vi "Simulate Statechart.vi"(4 "C DLL path":path=path "D:/Users/jjensen/workspace/Simulated iRobot Navigation/Release/libSimulated iRobot Navigation.dll", 6 "Execution Mode":T12, 8 "stop":bool, 11 "Statechart Inputs In":T2={"net distance (mm)"=0, "net angle (deg)"=0, "Max Wheel Speed (mm/s)"=0, "accelerometer"={"x axis (g)"=0.0, "y axis (g)"=0.0, "z axis (g)"=0.0}, "iRobot Sensors"={"Bumps + Wheel Drops"={"Wheeldrop Caster"=FALSE, "Wheeldrop Left"=FALSE, "Wheeldrop Right"=FALSE, "Bump Left"=FALSE, "Bump Right"=FALSE}, "Wall"=FALSE, "Cliff Left"=FALSE, "Cliff Front Left"=FALSE, "Cliff Front Right"=FALSE, "Cliff Right"=FALSE, "Virtual Wall"=FALSE, "Low-Side Driver + Wheel Overcurrent"={"Low-Side Driver 0"=FALSE, "Low-Side Driver 1"=FALSE, "Low-Side Driver 2"=FALSE, "Left Wheel"=FALSE, "Right Wheel"=FALSE}, "Infrared"=255, "Buttons"={"Advance"=FALSE, "Play"=FALSE}, "Distance (mm)"=0, "Angle (deg)"=0, "Charging State"=enum."Not Charging", "Voltage (mV)"=0, "Current (mA)"=0, "Battery Temperature (deg C)"=0, "Battery Charge (mAh)"=0, "Battery Capacity (mAh)"=0, "Wall Signal (0-4095)"=0, "Cliff Left Signal (0-4095)"=0, "Cliff Front Left Signal (0-4095)"=0, "Cliff Front Right Signal (0-4095)"=0, "Cliff Right Signal (0-4095)"=0, "Cargo Bay Digital Inputs"={"Digital Input 0"=FALSE, "Digital Input 1"=FALSE, "Digital Input 2"=FALSE, "Digital Input 3"=FALSE, "Device Detect"=FALSE}, "Cargo Bay Analog Signal (0-1023)"=0, "Charging Sources Available"={"Internal Charger"=FALSE, "Home Base"=FALSE}, "OI Mode"=enum."Off", "Song Number"=0, "Song Playing"=FALSE, "Number of Stream Packets"=0, "Requested Velocity (mm/s)"=0, "Requested Radius (mm)"=0, "Requested Right Wheel Velocity (mm/s)"=0, "Requested Left Wheel Velocity (mm/s)"=0}, "Is Simulator?"=FALSE} {"iRobot Sensors"."Infrared" format="%02x"; "accelerometer"."z axis (g)" format="%.3f"; "accelerometer"."y axis (g)" format="%.3f"; "accelerometer"."x axis (g)" format="%.3f"; "Max Wheel Speed (mm/s)" scale=0.0..500.0}) -> (0 "Left Wheel Speed (mm/s)":i16, 1 "Right Wheel Speed (mm/s)":i16, 2 "Diagram Display":picture, 3 "Statechart Inputs Out":T2={"net distance (mm)"=0, "net angle (deg)"=0, "Max Wheel Speed (mm/s)"=0, "accelerometer"={"x axis (g)"=0.0, "y axis (g)"=0.0, "z axis (g)"=0.0}, "iRobot Sensors"={"Bumps + Wheel Drops"={"Wheeldrop Caster"=FALSE, "Wheeldrop Left"=FALSE, "Wheeldrop Right"=FALSE, "Bump Left"=FALSE, "Bump Right"=FALSE}, "Wall"=FALSE, "Cliff Left"=FALSE, "Cliff Front Left"=FALSE, "Cliff Front Right"=FALSE, "Cliff Right"=FALSE, "Virtual Wall"=FALSE, "Low-Side Driver + Wheel Overcurrent"={"Low-Side Driver 0"=FALSE, "Low-Side Driver 1"=FALSE, "Low-Side Driver 2"=FALSE, "Left Wheel"=FALSE, "Right Wheel"=FALSE}, "Infrared"=255, "Buttons"={"Advance"=FALSE, "Play"=FALSE}, "Distance (mm)"=0, "Angle (deg)"=0, "Charging State"=enum."Not Charging", "Voltage (mV)"=0, "Current (mA)"=0, "Battery Temperature (deg C)"=0, "Battery Charge (mAh)"=0, "Battery Capacity (mAh)"=0, "Wall Signal (0-4095)"=0, "Cliff Left Signal (0-4095)"=0, "Cliff Front Left Signal (0-4095)"=0, "Cliff Front Right Signal (0-4095)"=0, "Cliff Right Signal (0-4095)"=0, "Cargo Bay Digital Inputs"={"Digital Input 0"=FALSE, "Digital Input 1"=FALSE, "Digital Input 2"=FALSE, "Digital Input 3"=FALSE, "Device Detect"=FALSE}, "Cargo Bay Analog Signal (0-1023)"=0, "Charging Sources Available"={"Internal Charger"=FALSE, "Home Base"=FALSE}, "OI Mode"=enum."Off", "Song Number"=0, "Song Playing"=FALSE, "Number of Stream Packets"=0, "Requested Velocity (mm/s)"=0, "Requested Radius (mm)"=0, "Requested Right Wheel Velocity (mm/s)"=0, "Requested Left Wheel Velocity (mm/s)"=0}, "Is Simulator?"=FALSE} {"iRobot Sensors"."Infrared" format="%02x"; "accelerometer"."z axis (g)" format="%.3f"; "accelerometer"."y axis (g)" format="%.3f"; "accelerometer"."x axis (g)" format="%.3f"; "Max Wheel Speed (mm/s)" scale=0.0..500.0}, 5 "Active States":string[](array[string]))   [LabVIEW 2013]
uses:
  Simulate Execution Mode.ctl
  iRobot Navigation State Machine.lvsc/Inputs.ctl
  Accelerometer.ctl
  iRobot/Sensor/Sensor Group 6.ctl
  iRobot/Sensor/Bumps + Wheel Drops.ctl
  iRobot/Sensor/Low-Side Driver + Wheel Overcurrent.ctl
  iRobot/Sensor/Buttons.ctl
  iRobot/Sensor/Charging State.ctl
  iRobot/Sensor/Cargo Bay Digital Inputs.ctl
  iRobot/Sensor/Charging Sources Available.ctl
  iRobot/Sensor/OI Mode.ctl
  iRobot Navigation State Machine.lvsc/StatechartState.ctl
  iRobot Navigation State Machine.lvsc/State.ctl
  iRobot Navigation State Machine.lvsc/CompanionDiagram.vi/64/SC Main.vi
  iRobot Navigation State Machine.lvsc/CompanionDiagram.vi/64/Upd State.vi
  iRobot Navigation State Machine.lvsc/CompanionDiagram.vi/64/Trans Graph0.vi
  iRobot Navigation State Machine.lvsc/CompanionDiagram.vi/64/EnterGraphCore.vi
  iRobot Navigation State Machine.lvsc/CompanionDiagram.vi/64/Trans Graph1.vi
  iRobot Navigation State Machine.lvsc/CompanionDiagram.vi/64/Trans Graph2.vi
  iRobot Navigation State Machine.lvsc/CompanionDiagram.vi/64/Trans Graph3.vi
  <vilib>/Analysis/coordinate.llb/Wrap Angle.vi
  <vilib>/Analysis/coordinate.llb/Wrap Angle (scalar).vi
  iRobot Navigation State Machine.lvsc/CompanionDiagram.vi
  Hamming Distance.vi
  Create Message.vi
  Process Message.vi
  Select.vi
  Wheel Speed Filter.vi
  iRobot Navigation State Machine.lvsc/Trigger.ctl
  <vilib>/Statechart/Infrastructure/RTStatechart/RunTime SCN.xnode
  iRobot Navigation State Machine.lvsc/Outputs.ctl
  iRobot Navigation State Machine.lvsc
panel:
  out "Bytes Written Last":i32
  out "Hamming Distance":u32
  out "Parent Display":T1(plugin-control)
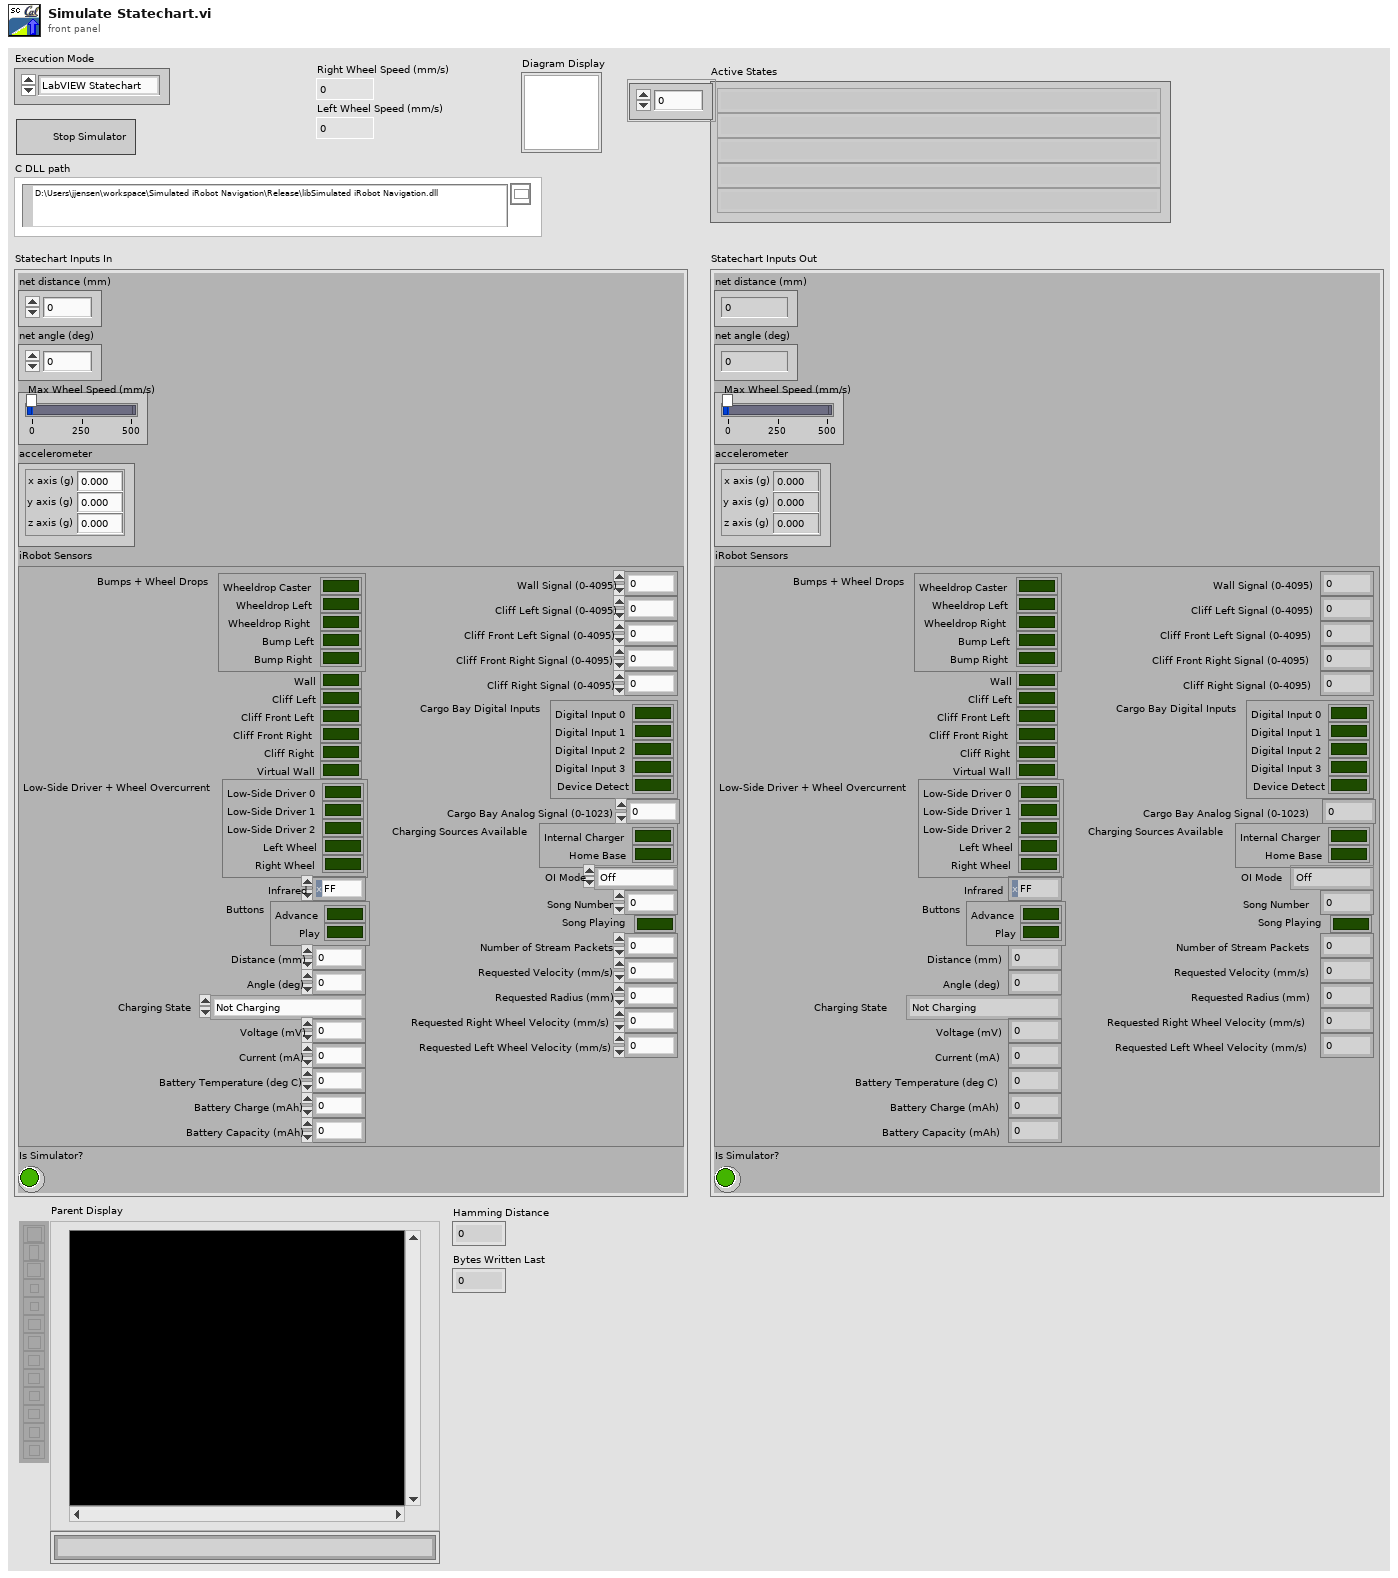
[diagram p1: front panel]
types:
  T1 = typedef "IMAQ Image.ctl" = refnum<image>
  T2 = typedef "iRobot Navigation State Machine.lvsc/Inputs.ctl" = cluster{"net distance (mm)":i32, "net angle (deg)":i32, "Max Wheel Speed (mm/s)":i16, "accelerometer":T3, "iRobot Sensors":T4, "Is Simulator?":bool}
  T3 = typedef "Accelerometer.ctl" = cluster{"x axis (g)":dbl, "y axis (g)":dbl, "z axis (g)":dbl}
  T4 = typedef "Sensor Group 6.ctl" = cluster{"Bumps + Wheel Drops":T5, "Wall":bool, "Cliff Left":bool, "Cliff Front Left":bool, "Cliff Front Right":bool, "Cliff Right":bool, "Virtual Wall":bool, "Low-Side Driver + Wheel Overcurrent":T6, "Infrared":u8, "Buttons":T7, "Distance (mm)":i32, "Angle (deg)":i32, "Charging State":T8, "Voltage (mV)":u16, "Current (mA)":i16, "Battery Temperature (deg C)":i8, "Battery Charge (mAh)":u16, "Battery Capacity (mAh)":u16, "Wall Signal (0-4095)":u16, "Cliff Left Signal (0-4095)":u16, "Cliff Front Left Signal (0-4095)":u16, "Cliff Front Right Signal (0-4095)":u16, "Cliff Right Signal (0-4095)":u16, "Cargo Bay Digital Inputs":T9, "Cargo Bay Analog Signal (0-1023)":u16, "Charging Sources Available":T10, "OI Mode":T11, "Song Number":u8, "Song Playing":bool, "Number of Stream Packets":u8, "Requested Velocity (mm/s)":i16, "Requested Radius (mm)":i16, "Requested Right Wheel Velocity (mm/s)":i16, "Requested Left Wheel Velocity (mm/s)":i16}
  T5 = typedef "Bumps + Wheel Drops.ctl" = cluster{"Wheeldrop Caster":bool, "Wheeldrop Left":bool, "Wheeldrop Right":bool, "Bump Left":bool, "Bump Right":bool}
  T6 = typedef "Low-Side Driver + Wheel Overcurrent.ctl" = cluster{"Low-Side Driver 0":bool, "Low-Side Driver 1":bool, "Low-Side Driver 2":bool, "Left Wheel":bool, "Right Wheel":bool}
  T7 = typedef "Buttons.ctl" = cluster{"Advance":bool, "Play":bool}
  T8 = typedef "Charging State.ctl" = enum16{"Not Charging", "Reconditioning Charging", "Full Charging", "Trickle Charging", "Waiting", "Charging Fault Condition"}
  T9 = typedef "Cargo Bay Digital Inputs.ctl" = cluster{"Digital Input 0":bool, "Digital Input 1":bool, "Digital Input 2":bool, "Digital Input 3":bool, "Device Detect":bool}
  T10 = typedef "Charging Sources Available.ctl" = cluster{"Internal Charger":bool, "Home Base":bool}
  T11 = typedef "OI Mode.ctl" = enum16{"Off", "Passive", "Safe", "Full"}
  T12 = typedef "Simulate Execution Mode.ctl" = enum16{"LabVIEW Statechart", "C Statechart"}
  T13 = typedef "iRobot Navigation State Machine.lvsc/StatechartState.ctl" = T14[]
  T14 = typedef "iRobot Navigation State Machine.lvsc/State.ctl" = enum16{"NI.SC.Initial", "NI.SC.History", "NI.SC.ShallowHistory", "NI.SC.Terminal", "End", "Running", "Start", "Running\\NI.SC.UnnamedRegion 0\\Genetic Algorithm", "Running\\NI.SC.UnnamedRegion 0\\Detect Collision", "Running\\NI.SC.UnnamedRegion 0\\Move Around", "Running\\NI.SC.UnnamedRegion 0\\Update LED", "Running\\NI.SC.UnnamedRegion 0\\Genetic Algorithm\\NI.SC.UnnamedRegion 0\\Determine\nNew Parent", "Running\\NI.SC.UnnamedRegion 0\\Genetic Algorithm\\NI.SC.UnnamedRegion 0\\Transfer Runnersup", "Running\\NI.SC.UnnamedRegion 0\\Genetic Algorithm\\NI.SC.UnnamedRegion 0\\Select Best", "Running\\NI.SC.UnnamedRegion 0\\Genetic Algorithm\\NI.SC.UnnamedRegion 0\\Get Other Parent", "Running\\NI.SC.UnnamedRegion 0\\Move Around\\NI.SC.UnnamedRegion 0\\Back Up", "Running\\NI.SC.UnnamedRegion 0\\Move Around\\NI.SC.UnnamedRegion 0\\Turn", "Running\\NI.SC.UnnamedRegion 0\\Move Around\\NI.SC.UnnamedRegion 0\\Drive"}
  T15 = typedef "iRobot Navigation State Machine.lvsc/Outputs.ctl" = cluster{"Left Wheel Speed (mm/s)":i16, "Right Wheel Speed (mm/s)":i16, "Parent":u8[], "Hamming Dist":u32, "Last Bytes Written":i32, "TCP Error":errorcluster}
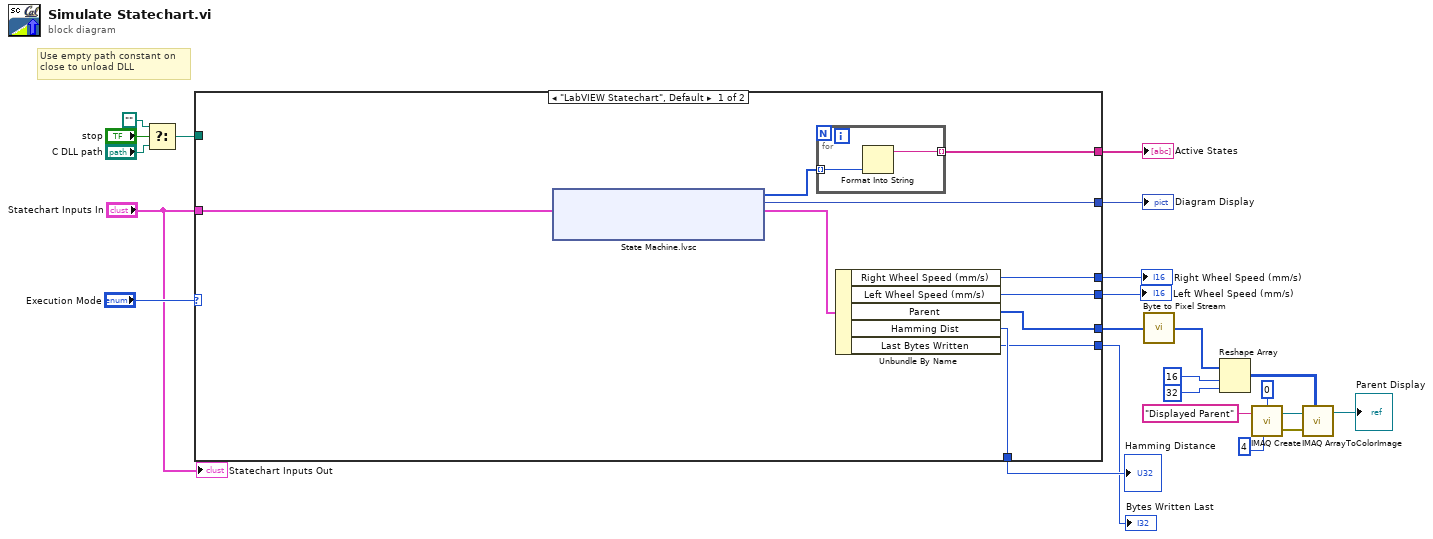
[diagram p0: block diagram]
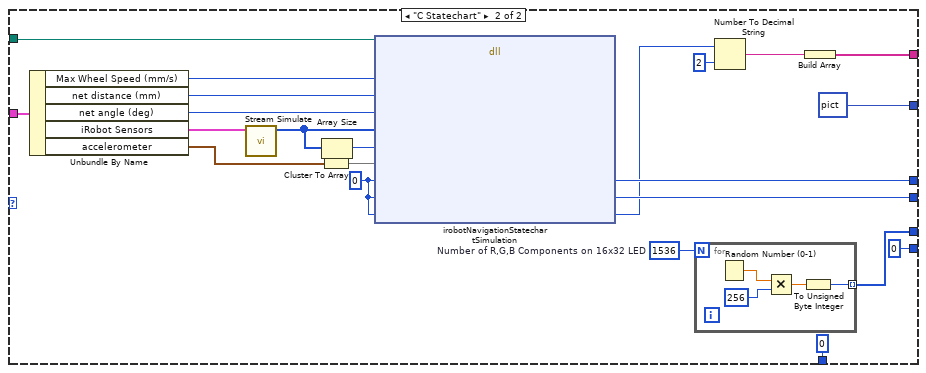
[diagram p2: hidden frame]
diagram:
  # "Use empty path constant on\nclose to unload DLL"
  n1 = Select(t=path "", s="stop", f="C DLL path") -> (s? t:f=w21:path)
  n2 = case shown="\"LabVIEW Statechart\", Default" "Execution Mode" {
    tunnel: w21 -> [_ w196]
    tunnel: [w32 w193] -> w19
    tunnel: [w31 w192] -> w18
    tunnel: [w30 picture data[5B] ("Diagram Display")] -> w16
    tunnel: [w27 w182] -> w14
    tunnel: "Statechart Inputs In" -> [w29 w190]
    tunnel: [w26 w177] -> w4
    tunnel: [w25 u32 0 ("Hamming Dist")] -> w2
    tunnel: [w24 0 ("Last Bytes Written")] -> w1
    frame "LabVIEW Statechart", Default {
      n3 = xnode ("State Machine.lvsc")("Inputs"=w29) -> ("Outputs"=w33:T15, "Active States"=w28:T13, "Diagram Display"=w30:picture)  [unwired: 3 in, 1 out]
      n4 = for {
        tunnel: w28 -> [w35] mode=indexing
        tunnel: [w34] -> w27 mode=indexing
        n5 = Format Into String(w35) -> (resulting string=w34:string)  [unwired: 3 in, 1 out]
      }
      n6 = Unbundle By Name(w33) -> ("Right Wheel Speed (mm/s)"=w32:i16, "Left Wheel Speed (mm/s)"=w31:i16, "Parent"=w26:u8[], "Hamming Dist"=w25:u32, "Last Bytes Written"=w24:i32)
    }
    frame "C Statechart" {
      w178 = 1536  # Number of R,G,B Components on 16x32 LED
      w183 = i16 0 ("rightWheelSpeed")
      n7 = Unbundle By Name(w190) -> ("Max Wheel Speed (mm/s)"=w189:i16, "net distance (mm)"=w188:i32, "net angle (deg)"=w187:i32, "iRobot Sensors"=w186:T4, "accelerometer"=w185:T3)
      n8 = call "Stream Simulate.vi"("iRobot Sensor Group 6"=w186) -> ("stream"=w194:u8[])  [unwired: 9 in, 1 out]
      n9 = Cluster To Array(cluster=w185) -> (array=w184:dbl[])
      n10 = Array Size(array=w194) -> (size(s)=w195:i32)
      n11 = dll-call lib="D:/Users/jjensen/workspace/Simulated iRobot Navigation/Release/libSimulated iRobot Navigation.dll" fn="irobotNavigationStatechartSimulation"(path in=w196, "wheelSpeed"=w189, "netDistance"=w188, "netAngle"=w187, "sensorStream"=w194, "sensorStreamSize"=w195, "accelAxes"=w184, "rightWheelSpeed"=w183, "leftWheelSpeed"=w183, "state"=w183) -> ("rightWheelSpeed"=w193:i16, "leftWheelSpeed"=w192:i16, "state"=w181:i32)  [unwired: 9 in, 2 out]
      n12 = for {
        N: w178 -> [_]
        tunnel: [w197] -> w177 mode=indexing
        n13 = Random Number (0-1)() -> (number: 0 to 1=w200:dbl)
        n14 = Multiply(x=w200, y=256) -> (x*y=w198:dbl)
        n15 = To Unsigned Byte Integer(number=w198) -> (unsigned 8bit integer=w197:u8)
      }
      n16 = Number To Decimal String(number=w181, width (-)=i16 2) -> (decimal integer string=w180:string)
      n17 = Build Array(w180) -> (w182:string[])
    }
  }
  "Right Wheel Speed (mm/s)" <- w19
  "Left Wheel Speed (mm/s)" <- w18
  "Diagram Display" <- w16
  "Active States" <- w14
  "Hamming Distance" <- w2
  "Bytes Written Last" <- w1
  n18 = call "Byte to Pixel Stream.vi"("RGB Byte Stream"=w4) -> ("Pixel Stream"=w3:u32[])
  n19 = Reshape Array(w3, 16 ("Constant"), 32 ("Constant 2")) -> (w11:u32[][])
  n20 = call "IMAQ Create"("Border Size"=0 ("Constant 4"), "Image Name"="Displayed Parent" ("Constant 3"), "Image Type"=4 ("Constant 5")) -> ("New Image"=w10:T1, "error out"=w9:errorcluster)  [unwired: 2 in]
  n21 = call "IMAQ ArrayToColorImage"("Image Pixels (U32)"=w11, "Image"=w10, "error in (no error)"=w9) -> ("Image Out"=→"Parent Display":T1)  [unwired: 2 in, 1 out]
  "Statechart Inputs Out" <- "Statechart Inputs In"
